vi "Array Size.vi"(0 "Controller Array in":refnum<class "Controller Array.lvclass">, 1 "error in (no error)":errorcluster) -> (2 "Controller Array out":refnum<class "Controller Array.lvclass">, 3 "size(s)":i32, 4 "error out":errorcluster)   [LabVIEW 2020, in "RxnRover.lvlib" / "Controller Array.lvclass"]
uses:
  Controller Array.lvclass
  Controller Array.lvclass/Controller Array.ctl
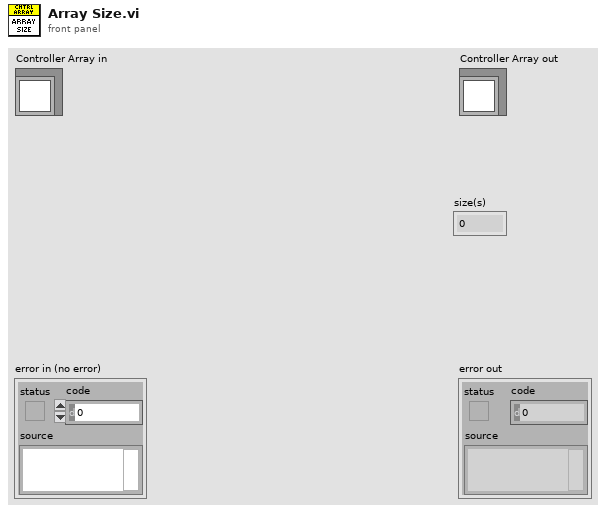
[diagram p1: front panel]
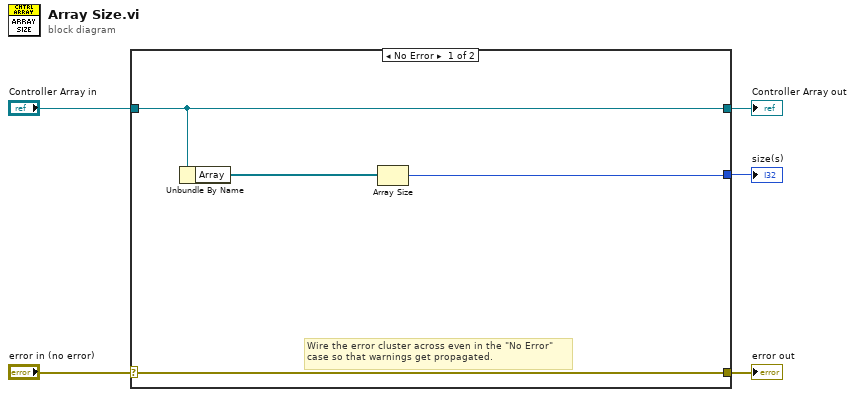
[diagram p0: block diagram]
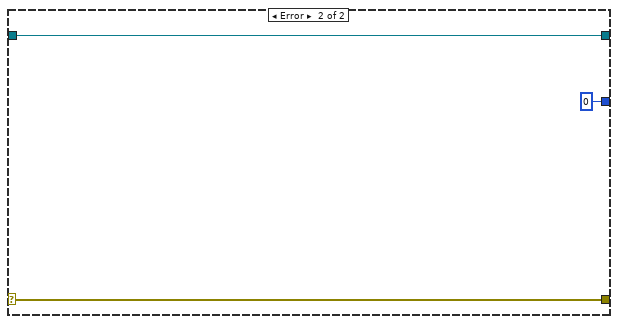
[diagram p2: hidden frame]
diagram:
  n1 = case shown="No Error" "error in (no error)" {
    selector: "error in (no error)" -> [w9 w12]
    tunnel: [w9 w12] -> w4
    tunnel: [w8 w11] -> w2
    tunnel: "Controller Array in" -> [w8 w11]
    tunnel: [w6 0] -> w1
    frame No Error {
      # "Wire the error cluster across even in the \"No Error\"\ncase so that warnings get propagated."
      n2 = Unbundle By Name(w8) -> ("Array"=w7:refnum<class "Generic Plugin.lvclass">[])
      n3 = Array Size(array=w7) -> (size(s)=w6:i32)
    }
    frame Error {
    }
  }
  "error out" <- w4
  "Controller Array out" <- w2
  "size(s)" <- w1
